vi "Insert.vi"(6 "Item":T1={"Item offset"=-1, "Offset past Item"=-1, "Name offset"=-1, "Offset past Name"=-1, "Found"=FALSE, "Item Type"=enum."Parser Error", "Item Index"=-1, "Start Offset"=0, "Comma Needed For Insert"=enum."False"}, 9 "<JSON>name":string, 10 "JSON to Insert":string, 11 "JSON in":string) -> (1 "Inserted Item Offset":i32, 2 "Found":bool, 3 "string":string)   [LabVIEW 2020, in "JSONtext.lvlib"]
uses:
  <vilib>/JDP Science/JSONtext/JSONtext.lvlib
  <vilib>/JDP Science/JSONtext/Parsing/Found Items.ctl
  <vilib>/JDP Science/JSONtext/Parsing/Parsing State.ctl
  <vilib>/JDP Science/JSONtext/support/Comma Needed for Insert.ctl
  <vilib>/JDP Science/JSONtext/Parsing/Advance past replacable whitespace.vi
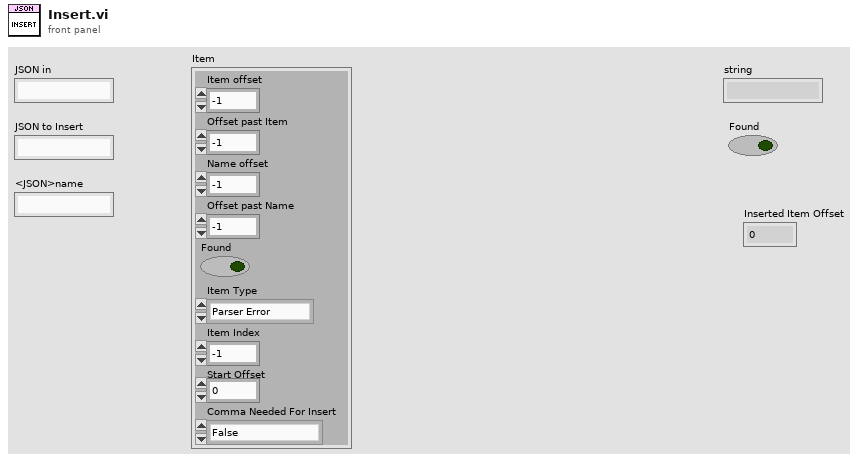
[diagram p1: front panel]
types:
  T1 = typedef "JSONtext.lvlib/Found Items.ctl" = cluster{"Item offset":i32, "Offset past Item":i32, "Name offset":i32, "Offset past Name":i32, "Found":bool, "Item Type":T2, "Item Index":i32, "Start Offset":i32, "Comma Needed For Insert":T3}
  T2 = typedef "JSONtext.lvlib/Parsing State.ctl" = enum16{"Parser Error", "Object", "Array", "String", "Number/Other", "Leading Whitespace", "Object end", "Array end", "Value end"}
  T3 = typedef "JSONtext.lvlib/Comma Needed for Insert.ctl" = enum8{"False", "True", "Following"}
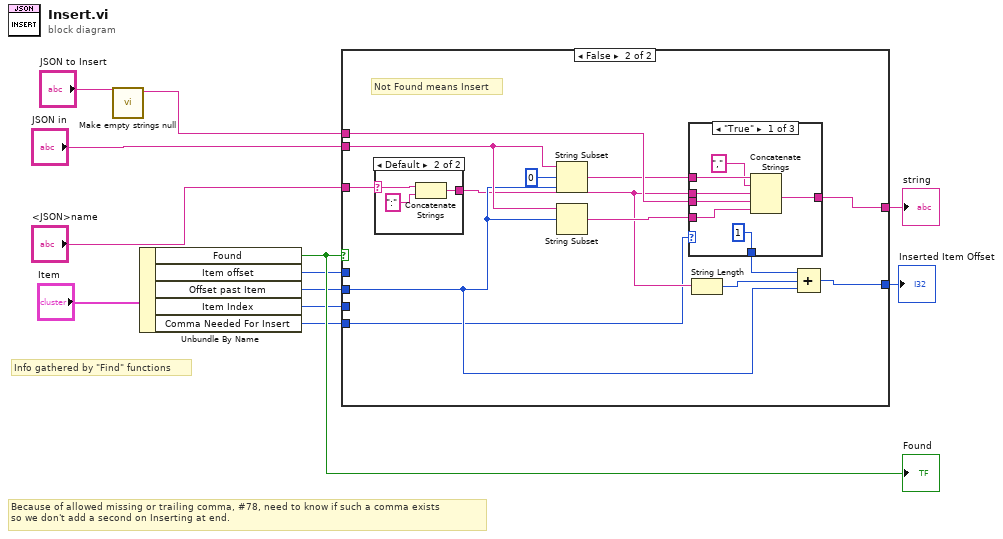
[diagram p0: block diagram]
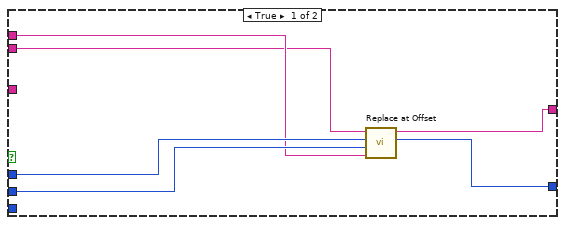
[diagram p2: hidden frame]
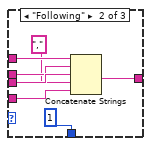
[diagram p3: hidden frame]
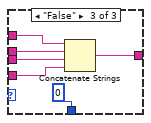
[diagram p4: hidden frame]
diagram:
  # "Info gathered by \"Find\" functions"
  # "Because of allowed missing or trailing comma, #78, need to know if such a comma exists \nso we don't add a second on Inserting at end."
  n1 = call <vilib>:"Make empty strings null.vi"("JSON Input"="JSON to Insert") -> ("<JSON>"=w2:string)  [unwired: 10 in]
  n2 = Unbundle By Name("Item") -> ("Found"=w11:bool, "Item offset"=w8:i32, "Offset past Item"=w7:i32, "Item Index"=w6:i32, "Comma Needed For Insert"=w1:T3)
  "Found" <- w11
  n3 = case shown="False" w11 {
    tunnel: "JSON in" -> [w14 w31]
    tunnel: w2 -> [w15 w30]
    tunnel: [w18 w29] -> w9
    tunnel: "<JSON>name" -> [_ w22]
    tunnel: w8 -> [w17 _]
    tunnel: w7 -> [w16 w23]
    tunnel: w6 -> [_ _]
    tunnel: [w13 w24] -> w4
    tunnel: w1 -> [_ w20]
    frame True {
      n4 = call <vilib>:"Replace at Offset.vi"("JSON to Insert"=w15, "Offset past Item"=w16, "Item offset"=w17, "<JSON> in"=w14) -> ("Item offset"=w13:i32, "<JSON>"=w18:string)  [unwired: 6 in]
    }
    frame False {
      # "Not Found means Insert"
      n5 = case shown="Default" w22 {
        selector: w22 -> [_ w53]
        tunnel: [_ w52] -> w21
        frame "" {
          # "Array insert"
        }
        frame Default {
          n6 = Concatenate Strings(w53, ":" ("string")) -> (w52:string)
        }
      }
      n7 = String Subset(string=w31, offset (0)=0 ("Value start in"), length (rest)=w23) -> (substring=w27:string)
      n8 = String Subset(string=w31, offset (0)=w23) -> (substring=w26:string)  [unwired: 1 in]
      n9 = case shown="\"True\"" w20 {
        tunnel: w30 -> [w38 w45 w51]
        tunnel: [w37 w44 w50] -> w29
        tunnel: w27 -> [w36 w43 w49]
        tunnel: w26 -> [w35 w42 w48]
        tunnel: w21 -> [w34 w41 w47]
        tunnel: [1 ("length") 1 ("length") 0 ("length")] -> w19
        frame "True" {
          n10 = Concatenate Strings(w36, "," ("string"), w34, w38, w35) -> (w37:string)
        }
        frame "Following" {
          n11 = Concatenate Strings(w43, w41, w45, "," ("string"), w42) -> (w44:string)
        }
        frame "False" {
          n12 = Concatenate Strings(w49, w47, w51, w48) -> (w50:string)
        }
      }
      n13 = String Length(string=w21) -> (length=w25:i32)
      n14 = Compound Arithmetic op=ADD(w19, w25, w23) -> (w24:i32)
    }
  }
  "string" <- w9
  "Inserted Item Offset" <- w4
